vi "FourCornerAntennaPositionToXYcoordinates.vi"() -> ()   [LabVIEW 2017]
doc: "This VI computes the x and y distance to move from antenna position 1 to position N.\nThen the subvi:\nOffsets those by the antenna Home (#1 position) to motion Home offset.\nCorrects for rotation of the antenna wrt the motion frame of ref."
panel:
  in  "x direction angle, deg":dbl=0.295 format="%#_13g"
  in  "y patch 1 position, mm":dbl=144.21 format="%#_13g"
  in  "x patch 1 position, mm":dbl=204.42 format="%#_13g"
  out "y":dbl=145.2088475177728
  out "x":dbl=398.41742860057764
  in  "Position, 1 - 64":dbl=8.0
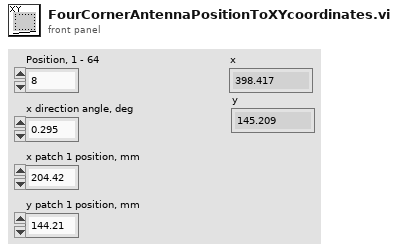
[diagram p1: front panel]
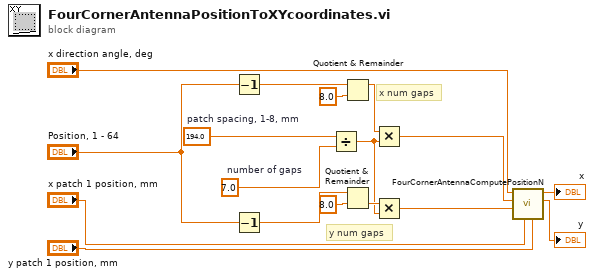
[diagram p0: block diagram]
diagram:
  w13 = 7.0  # number of gaps
  w14 = 194.0  # patch spacing, 1-8, mm
  # "x num gaps"
  # "y num gaps"
  n1 = Decrement(x="Position, 1 - 64") -> (x-1=w12:dbl)
  n2 = Decrement(x="Position, 1 - 64") -> (x-1=w9:dbl)
  n3 = Divide(x=w14, y=w13) -> (x/y=w5:dbl)
  n4 = Quotient & Remainder(x=w12, y=8.0) -> (x-y*floor(x/y)=w7:dbl)  [unwired: 1 out]
  n5 = Quotient & Remainder(x=w9, y=8.0) -> (floor(x/y)=w6:dbl)  [unwired: 1 out]
  n6 = Multiply(x=w7, y=w5) -> (x*y=w4:dbl)
  n7 = Multiply(x=w6, y=w5) -> (x*y=w3:dbl)
  n8 = call "FourCornerAntennaComputePositionN.vi"("y patch 1 position, mm"="y patch 1 position, mm", "x patch 1 position, mm"="x patch 1 position, mm", "y distance, mm"=w3, "x distance, mm"=w4, "x direction angle, deg"="x direction angle, deg") -> ("y"=→"y":dbl, "x"=→"x":dbl)  [unwired: 5 in]
